vi "Setup.vi"(0 "Scalar SA Path in":refnum<class "SA Abstract Path.lvclass">, 11 "error in (no error)":errorcluster) -> (4 "Scalar SA Path out":refnum<class "SA Abstract Path.lvclass">, 15 "error out":errorcluster)   [LabVIEW 2023, in "RFFixtureCharact.Public.lvlib" / "SA Abstract Path.lvclass"]
uses:
  SA Abstract Path.lvclass
  Scalar Path/Scalar Path.lvclass
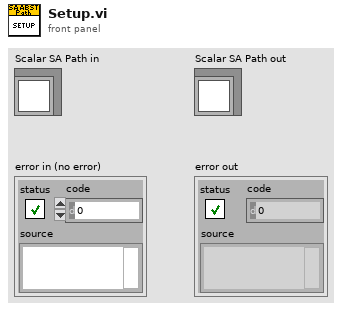
[diagram p1: front panel]
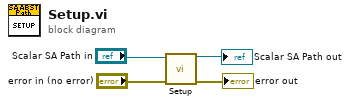
[diagram p0: block diagram]
diagram:
  n1 = call-parent "Setup.vi"("Scalar Path in"="Scalar SA Path in", "error in (no error)"="error in (no error)") -> ("Scalar Path out"=→"Scalar SA Path out":refnum<class "SA Abstract Path.lvclass">, "error out"=→"error out":errorcluster)  [unwired: 12 in]
